vi "Measure Time Elapsed.vi"(8 "Error In (no error)":errorcluster, 11 "VISA Resource Name":refnum<visa-resource-name>) -> (0 "Error Out":errorcluster, 2 "Time (0.0)":dbl format="%.2f", 3 "VISA Resource Name Out":refnum<visa-resource-name>)   [LabVIEW 2010, in "Stanford Research 844.lvlib"]
doc: "This VI measures the time elapsed."
uses:
  <instrlib>/Stanford Research 844/Stanford Research 844.lvlib
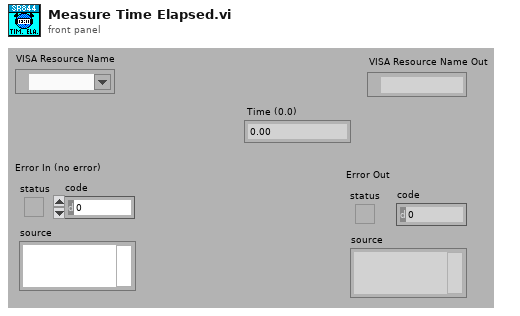
[diagram p1: front panel]
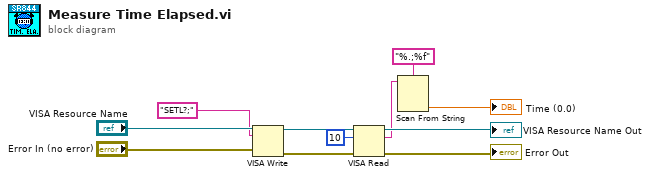
[diagram p0: block diagram]
diagram:
  n1 = VISA Write(VISA resource name="VISA Resource Name", write buffer="SETL?;" ("false string"), error in (no error)="Error In (no error)") -> (VISA resource name out=w11:refnum<visa-resource-name>, error out=w10:errorcluster)  [unwired: 1 out]
  n2 = VISA Read(VISA resource name=w11, byte count=u32 10 ("byte count (0)"), error in (no error)=w10) -> (VISA resource name out=→"VISA Resource Name Out":refnum<visa-resource-name>, read buffer=w3:string, error out=→"Error Out":errorcluster)  [unwired: 1 out]
  n3 = Scan From String(format string="%.;%f", input string=w3) -> (output 1=→"Time (0.0)":dbl)  [unwired: 3 in, 3 out]
